vi "Scan Engine Custom IO - From FPGA.vi"(8 "error in (no error)":errorcluster, 11 "Node Ptr":T1 format="%.0x") -> (0 "error out":errorcluster)   [LabVIEW 2016, in "Scan Engine Custom Device.lvlib"]
uses:
  Scan Engine Custom Device.lvlib
  <vilib>/NI Veristand/Custom Device API/Custom Device Item Ref.ctl
  Type Defs/UDV Data Type.ctl
  Type Defs/FXP Config.ctl
  Globals/Property Strings.vi
  <vilib>/NI Veristand/Custom Device API/Get Item Property (String).vi
  <vilib>/NI Veristand/Custom Device API/Get Item Property (U16).vi
  <vilib>/NI Veristand/Custom Device API/Get Item Property (Variant).vi
  <vilib>/NI Veristand/Custom Device API/Custom Device API.lvlib
panel:
  out "IO Variable Name":string
  in  "Units":string
  out "Data Type":string
  in  "Header":cluster{"Section Name":string}={"Section Name"="Custom FPGA I/O"}
  in  "Description":string
  in  "Name":string
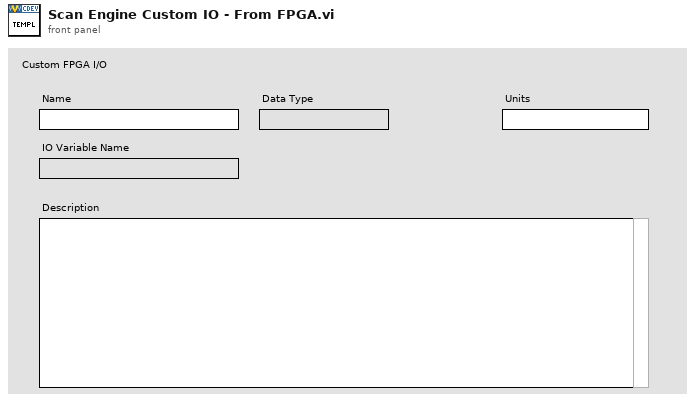
[diagram p1: front panel]
types:
  T1 = typedef "Custom Device API.lvlib/Custom Device Item Ref.ctl" = u64
  T2 = typedef "Scan Engine Custom Device.lvlib/UDV Data Type.ctl" = enum16{"Boolean", "Fixed Point", "Int8", "Int16", "Int32", "Int64", "U32 Bit Field", "UInt8", "UInt16", "UInt32", "UInt64", "Other"}
  T3 = typedef "Custom Device API.lvlib/Custom Device Item Info.ctl" = cluster{"Name":string, "Is Channel":bool, "GUID":string, "Is Waveform":bool}
  T4 = typedef "Custom Device API.lvlib/Custom Device Channel.ctl" = cluster{"Type":T5, "Units":string, "Default Value":dbl, "Faultable":bool, "Scalable":bool}
  T5 = typedef "Custom Device API.lvlib/Custom Device Channel Type.ctl" = enum16{"Input", "Output"}
  T6 = typedef "Scan Engine Custom Device.lvlib/FXP Config.ctl" = cluster{"signed":bool, "size":u32, "integersize":i32}
  T7 = typedef "Custom Device API.lvlib/Custom Device Commands.ctl" = enum16{"Default", "Item renamed", "Shutdown", "Dynamic button pressed"}
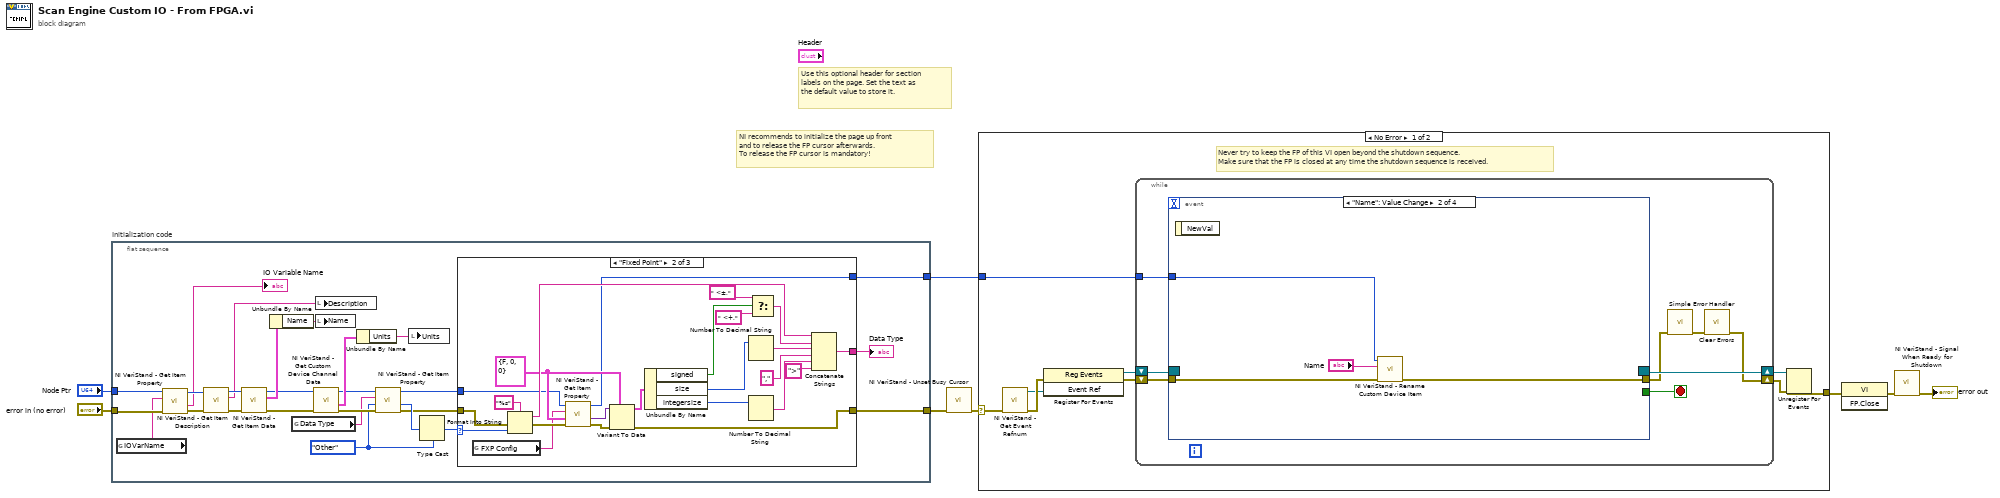
[diagram p0: block diagram]
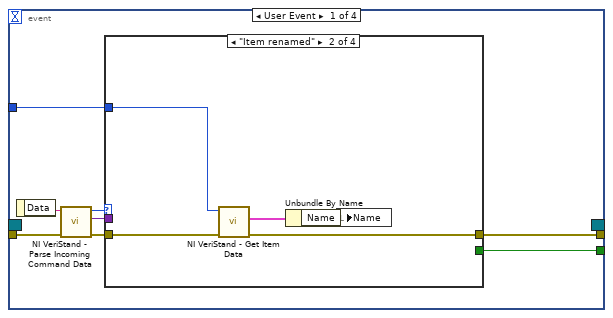
[diagram p2: hidden frame]
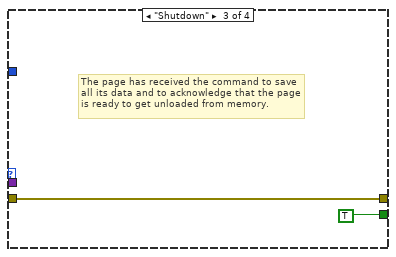
[diagram p4: hidden frame]
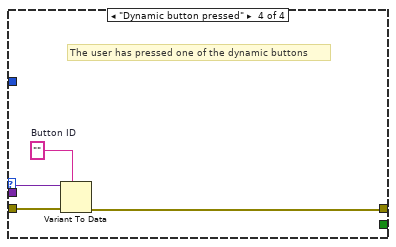
[diagram p5: hidden frame]
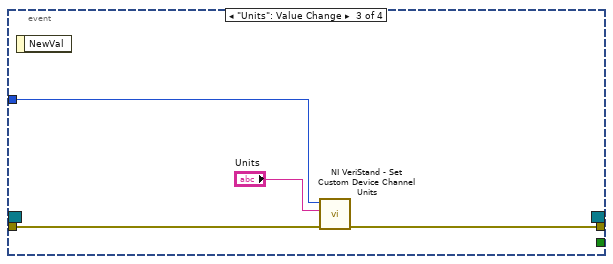
[diagram p6: hidden frame]
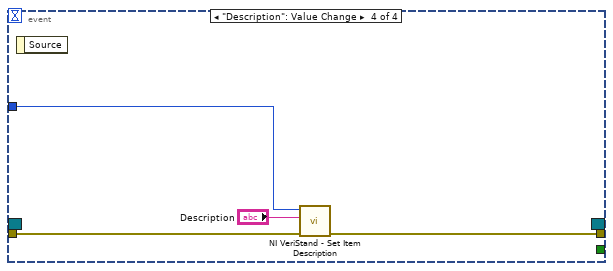
[diagram p7: hidden frame]
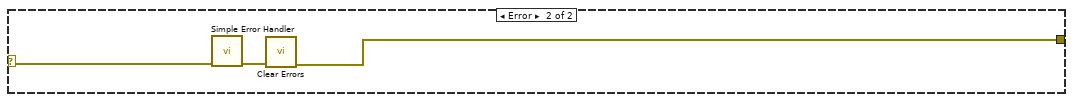
[diagram p8: hidden frame]
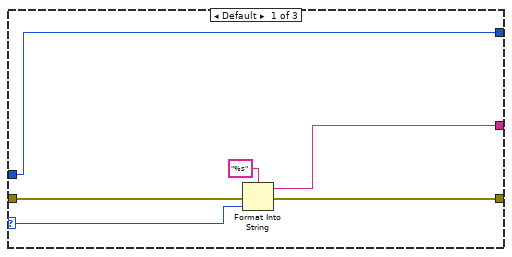
[diagram p9: hidden frame]
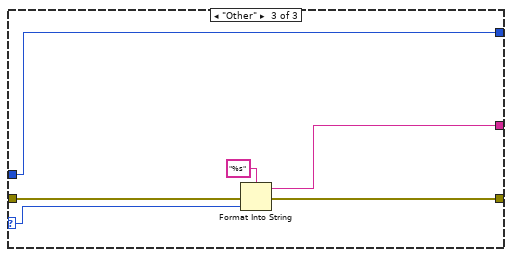
[diagram p10: hidden frame]
diagram:
  # "Use this optional header for section labels on the page. Set the text as the default value to store it."
  # "NI recommends to initialize the page up front\nand to release the FP cursor afterwards.\nTo release the FP cursor is mandatory!"
  n1 = flat-sequence "Initialization code" {
    tunnel: "error in (no error)" -> [w14]
    tunnel: "Node Ptr" -> [w13]
    tunnel: [w17] -> w4
    tunnel: [w15] -> w1
    frame #0 {
      w21 = UDV_Data_Type."Other" ("UDV Data Type out")
      n2 = global read "Property Strings.vi" "IOVarName"() -> (w10:string)
      n3 = call-poly <vilib>:"NI VeriStand - Get Item Property.vi"("error in (no error)"=w14, "Property Name"=w10, "Item Ref in"=w13) -> ("error out"=w11:errorcluster, "Value"=→"IO Variable Name":string, "Item Ref out"=w12:T1)  [unwired: 5 in, 1 out]
      n4 = call <vilib>:"NI VeriStand - Get Item Description.vi"("error in (no error)"=w11, "Item Ref in"=w12) -> ("error out"=w32:errorcluster, "Description"=w33:string, "Item Ref out"=w34:T1)  [unwired: 7 out]
      n5 = call <vilib>:"NI VeriStand - Get Item Data.vi"("error in (no error)"=w32, "Item Ref in"=w34) -> ("error out"=w28:errorcluster, "Item Info"=w31:T3, "Item Ref out"=w29:T1)  [unwired: 7 out]
      n6 = Unbundle By Name(w31) -> ("Name"=w30:string)
      n7 = global read "Property Strings.vi" "Data Type"() -> (w23:string)
      n8 = call <vilib>:"NI VeriStand - Get Custom Device Channel Data.vi"("error in (no error)"=w28, "Channel Ref in"=w29) -> ("error out"=w24:errorcluster, "Channel"=w27:T4, "Channel Ref out"=w25:T1)  [unwired: 4 in, 3 out]
      n9 = local write "Description"(w33) -> ()
      n10 = local write "Name"(w30) -> ()
      n11 = Unbundle By Name(w27) -> ("Units"=w26:string)
      n12 = call-poly <vilib>:"NI VeriStand - Get Item Property.vi"("error in (no error)"=w24, "Default Value"=w21, "Property Name"=w23, "Item Ref in"=w25) -> ("error out"=w20:errorcluster, "Value"=w22:u16, "Item Ref out"=w18:T1)  [unwired: 4 in, 1 out]
      n13 = local write "Units"(w26) -> ()
      n14 = Type Cast(type=w21, x=w22) -> (*(type *) &x=w19:T2)
      n15 = case shown="\"Fixed Point\"" w19 {
        selector: w19 -> [w39 w46 w68]
        tunnel: w20 -> [w40 w45 w69]
        tunnel: [w37 w42 w66] -> w16
        tunnel: [w36 w43 w67] -> w17
        tunnel: w18 -> [w35 w44 w65]
        tunnel: [w35 w41 w65] -> w15
        frame Default {
          n16 = Format Into String(format string="%s", error in=w40, w39) -> (resulting string=w37:string, error out=w36:errorcluster)  [unwired: 1 in]
        }
        frame "Fixed Point" {
          w50 = T6 {"signed"=FALSE, "size"=0, "integersize"=0} ("FXP Config")
          n17 = global read "Property Strings.vi" "FXP Config"() -> (w47:string)
          n18 = Format Into String(format string="%s", error in=w45, w46) -> (resulting string=w56:string, error out=w58:errorcluster)  [unwired: 1 in]
          n19 = call-poly <vilib>:"NI VeriStand - Get Item Property.vi"("error in (no error)"=w58, "Default Value"=w50, "Property Name"=w47, "Item Ref in"=w44) -> ("error out"=w48:errorcluster, "Value"=w49:variant, "Item Ref out"=w41:T1)  [unwired: 4 in, 1 out]
          n20 = Variant To Data(error in=w48, type=w50, Variant=w49) -> (data=w51:T6, error out=w43:errorcluster)
          n21 = Unbundle By Name(w51) -> ("signed"=w52:bool, "size"=w59:u32, "integersize"=w60:i32)
          n22 = Number To Decimal String(number=w59) -> (decimal integer string=w61:string)  [unwired: 1 in]
          n23 = Number To Decimal String(number=w60) -> (decimal integer string=w63:string)  [unwired: 1 in]
          n24 = Select(t=" <±,", s=w52, f=" <+,") -> (s? t:f=w57:string)
          n25 = Concatenate Strings(w56, w57, w61, ",", w63, ">") -> (w42:string)
        }
        frame "Other" {
          n26 = Format Into String(format string="%s", error in=w69, w68) -> (resulting string=w66:string, error out=w67:errorcluster)  [unwired: 1 in]
        }
      }
      "Data Type" <- w16
    }
  }
  n27 = call <vilib>:"NI VeriStand - Unset Busy Cursor.vi"("error in (no error)"=w4) -> ("error out"=w3:errorcluster)  [unwired: 10 out]
  n28 = case shown="No Error" w3 {
    selector: w3 -> [w72 w122]
    tunnel: [w76 w120] -> w8
    tunnel: w1 -> [w71 _]
    frame No Error {
      # "Never try to keep the FP of this VI open beyond the shutdown sequence.\nMake sure that the FP is closed at any time the shutdown sequence is received."
      n29 = call <vilib>:"NI VeriStand - Get Event Refnum.vi"("error in (no error)"=w72) -> ("error out"=w79:errorcluster, "Event Ref"=w75:refnum<user-event>)  [unwired: 9 out]
      n30 = register-events(error in=w79, w75) -> (reference out=w73:refnum<event-registration>, error out=w74:errorcluster)  [unwired: 1 in]
      n31 = while {
        shift-right: [w81] -> w77
        shift-left: w74 -> [w86]
        shift-right: [w87] -> w78
        shift-left: w73 -> [w85]
        tunnel: w71 -> [w80]
        stop <- w84 stop-if-true
        n32 = event shown="[1] \"Name\": Value Change" {
          selector: w85 -> [_ _ _ _]
          dyn-events: [_ _ _ _] -> w87
          timeout: _ -> [_ _ _ _]
          tunnel: w86 -> [w95 w111 w115 w119]
          tunnel: [w91 _ _ _] -> w84
          tunnel: [w90 w110 w113 w118] -> w83
          tunnel: w80 -> [w88 w108 w112 w116]
          event User Event {
            n33 = event-data() -> ("Data"=w94:string)  [unwired: 1 out]
            n34 = call <vilib>:"NI VeriStand - Parse Incoming Command Data.vi"("error in (no error)"=w95, "Incoming data"=w94) -> ("error out"=w93:errorcluster, "Outgoing data"=w89:variant, "Action"=w92:T7)  [unwired: 7 out]
            n35 = case shown="\"Item renamed\"" w92 {
              tunnel: w93 -> [w96 w101 w102 w107]
              tunnel: [_ _ TRUE _] -> w91
              tunnel: [w96 w99 w102 w104] -> w90
              tunnel: w89 -> [_ _ _ w106]
              tunnel: w88 -> [_ w97 _ _]
              frame "Default", Default {
              }
              frame "Item renamed" {
                n36 = call <vilib>:"NI VeriStand - Get Item Data.vi"("error in (no error)"=w101, "Item Ref in"=w97) -> ("error out"=w99:errorcluster, "Item Info"=w100:T3)  [unwired: 8 out]
                n37 = Unbundle By Name(w100) -> ("Name"=w98:string)
                n38 = local write "Name"(w98) -> ()
              }
              frame "Shutdown" {
                # "The page has received the command to save all its data and to acknowledge that the page is ready to get unloaded from memory."
              }
              frame "Dynamic button pressed" {
                w105 = ""  # Button ID
                # "The user has pressed one of the dynamic buttons"
                n39 = Variant To Data(error in=w107, type=w105, Variant=w106) -> (error out=w104:errorcluster)  [unwired: 1 out]
              }
            }
          }
          event "Name": Value Change {
            n40 = event-data() -> ()  [unwired: 2 out]
            n41 = call <vilib>:"NI VeriStand - Rename Custom Device Item.vi"("error in (no error)"=w111, "New Name"="Name", "Item Ref in"=w108) -> ("error out"=w110:errorcluster)  [unwired: 1 in, 7 out]
          }
          event "Units": Value Change {
            n42 = event-data() -> ()  [unwired: 2 out]
            n43 = call <vilib>:"NI VeriStand - Set Custom Device Channel Units.vi"("error in (no error)"=w115, "Units"="Units", "Channel Ref in"=w112) -> ("error out"=w113:errorcluster)  [unwired: 7 in, 1 out]
          }
          event "Description": Value Change {
            n44 = event-data() -> ()  [unwired: 2 out]
            n45 = call <vilib>:"NI VeriStand - Set Item Description.vi"("error in (no error)"=w119, "Description"="Description", "Item Ref in"=w116) -> ("error out"=w118:errorcluster)  [unwired: 8 out]
          }
        }
        n46 = call <vilib>:"Simple Error Handler.vi"("error in (no error)"=w83) -> ("error out"=w82:errorcluster)  [unwired: 1 in, 7 out]
        n47 = call <vilib>:"Clear Errors.vi"("error in (no error)"=w82) -> ("error out"=w81:errorcluster)  [unwired: 1 in, 5 out]
      }
      n48 = Unregister For Events(event registration refnum=w78, error in=w77) -> (error out=w76:errorcluster)
    }
    frame Error {
      n49 = call <vilib>:"Simple Error Handler.vi"("error in (no error)"=w122) -> ("error out"=w121:errorcluster)  [unwired: 1 in, 7 out]
      n50 = call <vilib>:"Clear Errors.vi"("error in (no error)"=w121) -> ("error out"=w120:errorcluster)  [unwired: 1 in, 5 out]
    }
  }
  n51 = invoke class="VI" method="FP.Close"(error in=w8) -> (error out=w7:errorcluster)  [unwired: 2 in, 2 out]
  n52 = call <vilib>:"NI VeriStand - Signal When Ready for Shutdown.vi"("error in (no error)"=w7) -> ("error out"=→"error out":errorcluster)  [unwired: 10 out]
